vi "encoder_test.vi"() -> ()   [LabVIEW 2011]
panel:
  in  "VISA COM IN":refnum<visa-resource-name>
  in  "stop":bool
  in  "Reset":bool
  out "Gauge":dbl(knob) scale=0.0..360.0
  # "Prueba básica de comunicación\ncon el Encoder del servomotor"
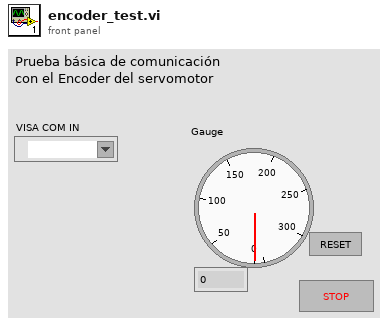
[diagram p1: front panel]
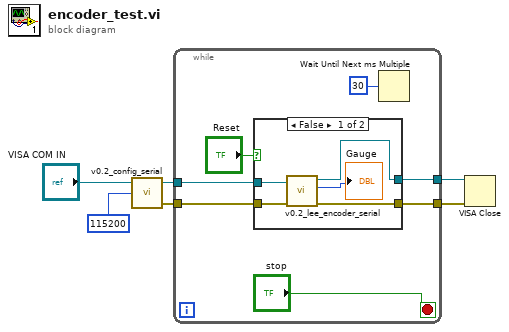
[diagram p0: block diagram]
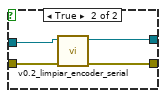
[diagram p2: hidden frame]
diagram:
  n1 = call "v0.2_config_serial.vi"("baud rate (9600/115200)"=u32 115200, "VISA COM IN"="VISA COM IN") -> ("error out"=w3:errorcluster, "VISA COM OUT"=w4:refnum<visa-resource-name>)  [unwired: 2 in]
  n2 = while {
    tunnel: w4 -> [w10]
    tunnel: w3 -> [w9]
    tunnel: [w8] -> w2
    tunnel: [w7] -> w1
    stop <- "stop" stop-if-true
    n3 = case shown="False" "Reset" {
      tunnel: w10 -> [w18 w22]
      tunnel: w9 -> [w17 w21]
      tunnel: [w16 w20] -> w8
      tunnel: [w15 w19] -> w7
      frame False {
        n4 = call "v0.2_lee_encoder_serial.vi"("error in (no error)"=w17, "VISA COM IN"=w18) -> ("error out"=w15:errorcluster, "grados"=→"Gauge":i32, "VISA COM OUT"=w16:refnum<visa-resource-name>)  [unwired: 7 in]
      }
      frame True {
        n5 = call "v0.2_limpiar_encoder_serial.vi"("error in (no error)"=w21, "VISA COM IN"=w22) -> ("error out"=w19:errorcluster, "VISA COM OUT"=w20:refnum<visa-resource-name>)  [unwired: 8 in]
      }
    }
    n6 = Wait Until Next ms Multiple(millisecond multiple=u32 30) -> ()  [unwired: 1 out]
  }
  n7 = VISA Close(VISA resource name=w2, error in (no error)=w1) -> ()  [unwired: 1 out]
